vi "ATS_Search_Value.vi"(4 "Search_Mode":enum16{"Extract", "Equal", "Closest"}(ring), 6 "Value In":dbl format="%.2f", 7 "StringArray":string[](array[string])=["1 kS/s", "2 kS/s", "5 kS/s", "10 kS/s", "20 kS/s", "50 kS/s", "100 kS/s", "200 kS/s", "500 kS/s", "1 MS/s", "2 MS/s", "5 MS/s", "10 MS/s", "20 MS/s", "25 MS/s", "50 MS/s", "100 MS/s", "200 MS/s", "500 MS/s", "1 GS/s"]) -> (1 "Index":i32, 2 "Out_Value":dbl format="%.2f", 3 "String":string)   [LabVIEW 2010]
doc: "_____AlazarTech, Scope_____\n\nSearch for closest Value IN if in the String Array and indicate is position.\nOut the value at the Value IN position in the String Array."
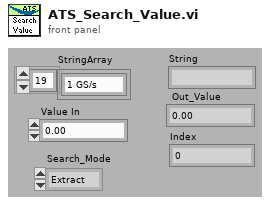
[diagram p1: front panel]
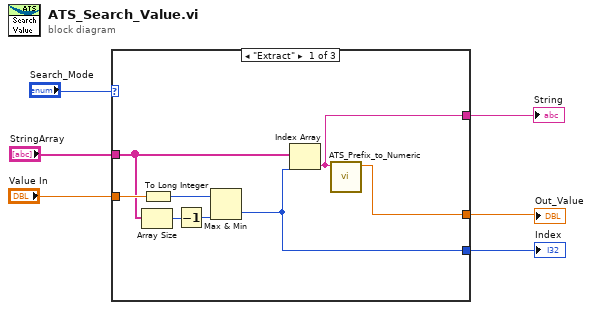
[diagram p0: block diagram]
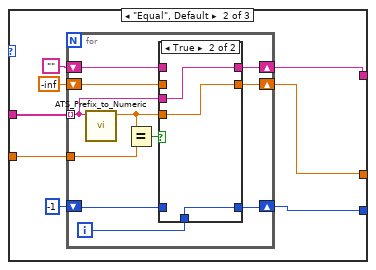
[diagram p2: hidden frame]
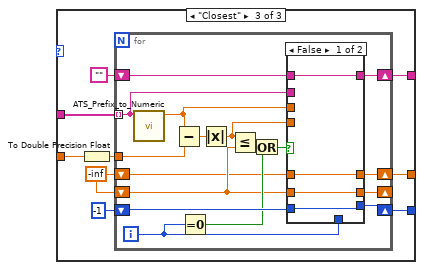
[diagram p4: hidden frame]
diagram:
  n1 = case shown="\"Extract\"" "Search_Mode" {
    tunnel: "Value In" -> [w14 w21 w47]
    tunnel: "StringArray" -> [w11 w22 w48]
    tunnel: [w7 w19 w45] -> w3
    tunnel: [w13 w17 w44] -> w1
    tunnel: [w12 w18 w43] -> w2
    frame "Extract" {
      n2 = Array Size(array=w11) -> (size(s)=w10:i32)
      n3 = To Long Integer(number=w14) -> (32bit integer=w8:i32)
      n4 = Decrement(x=w10) -> (x-1=w9:i32)
      n5 = Max & Min(x=w8, y=w9) -> (min(x,y)=w7:i32)  [unwired: 1 out]
      n6 = Index Array(array=w11, index=w7) -> (element=w12:string)
      n7 = call "ATS_Prefix_to_Numeric.vi"("String"=w12) -> ("Full Value"=w13:dbl)  [unwired: 4 in, 2 out]
    }
    frame "Equal", Default {
      n8 = for {
        shift-left: -1 -> [w32]
        shift-right: [w31] -> w19
        tunnel: w21 -> [w33]
        tunnel: w22 -> [w26] mode=indexing
        shift-right: [w27] -> w17
        shift-left: -inf -> [w23]
        shift-right: [w25] -> w18
        shift-left: "" -> [w24]
        i -> [w30]
        n9 = call "ATS_Prefix_to_Numeric.vi"("String"=w26) -> ("Full Value"=w28:dbl)  [unwired: 4 in, 2 out]
        n10 = Equal?(x=w28, y=w33) -> (x = y?=w29:bool)
        n11 = case shown="True" w29 {
          tunnel: w32 -> [w36 _]
          tunnel: [w36 w39] -> w31
          tunnel: w30 -> [_ w39]
          tunnel: w28 -> [_ w38]
          tunnel: [w34 w38] -> w27
          tunnel: w26 -> [_ w37]
          tunnel: [w35 w37] -> w25
          tunnel: w24 -> [w35 _]
          tunnel: w23 -> [w34 _]
          frame False {
          }
          frame True {
          }
        }
      }
    }
    frame "Closest" {
      w41 = -inf
      n12 = To Double Precision Float(number=w47) -> (double precision float=w40:dbl)
      n13 = for {
        shift-left: -1 -> [w64]
        shift-right: [w63] -> w45
        tunnel: w40 -> [w65]
        tunnel: w48 -> [w52] mode=indexing
        shift-right: [w54] -> w44
        shift-left: w41 -> [w53]
        shift-right: [w56] -> _
        shift-left: w41 -> [w55]
        shift-right: [w51] -> w43
        shift-left: "" -> [w50]
        i -> [w60]
        n14 = call "ATS_Prefix_to_Numeric.vi"("String"=w52) -> ("Full Value"=w57:dbl)  [unwired: 4 in, 2 out]
        n15 = Subtract(x=w57, y=w65) -> (x-y=w62:dbl)
        n16 = Equal To 0?(x=w60) -> (x = 0?=w59:bool)
        n17 = Absolute Value(x=w62) -> (abs(x)=w58:dbl)
        n18 = Less Or Equal?(x=w58, y=w55) -> (x <= y?=w61:bool)
        n19 = Or(x=w61, y=w59) -> (x .or. y?=w49:bool)
        n20 = case shown="False" w49 {
          tunnel: w64 -> [w67 _]
          tunnel: [w67 w73] -> w63
          tunnel: w60 -> [_ w73]
          tunnel: w58 -> [_ w72]
          tunnel: w57 -> [_ w71]
          tunnel: [w68 w72] -> w56
          tunnel: w55 -> [w68 _]
          tunnel: [w69 w71] -> w54
          tunnel: w53 -> [w69 _]
          tunnel: w52 -> [_ w70]
          tunnel: [w66 w70] -> w51
          tunnel: w50 -> [w66 _]
          frame False {
          }
          frame True {
          }
        }
      }
    }
  }
  "String" <- w2
  "Out_Value" <- w1
  "Index" <- w3
